vi "SetReference.vi"(8 "error in (no error)":errorcluster, 10 "Reference":string, 11 "Footnote in":refnum<class "FootnoteReference.lvclass">) -> (0 "error out":errorcluster, 3 "Footnote out":refnum<class "FootnoteReference.lvclass">)   [LabVIEW 2021, in "LvMarkdown.lvlib" / "FootnoteReference.lvclass"]
uses:
  FootnoteReference.lvclass
  FootnoteReference.lvclass/FootnoteReference.ctl
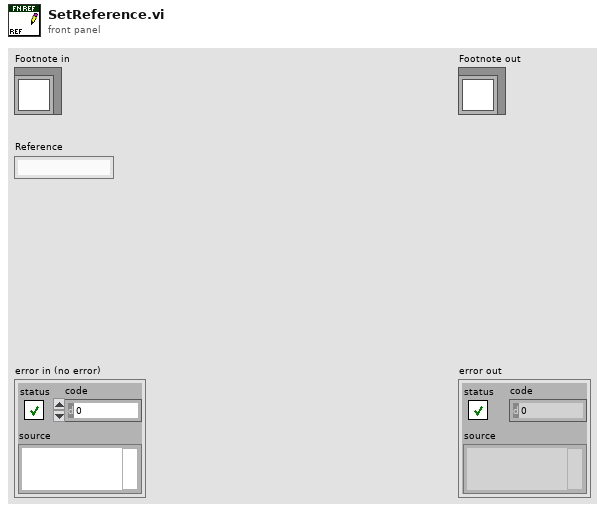
[diagram p1: front panel]
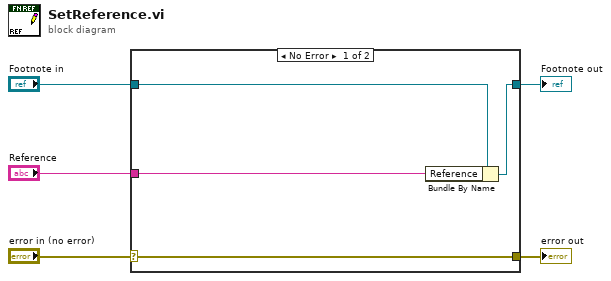
[diagram p0: block diagram]
diagram:
  n1 = case shown="No Error" "error in (no error)" {
    selector: "error in (no error)" -> [w9 w10]
    tunnel: [w9 w10] -> w4
    tunnel: [w7 w11] -> w2
    tunnel: "Footnote in" -> [w8 w11]
    tunnel: "Reference" -> [w6 _]
    frame No Error {
      n2 = Bundle By Name(cluster=w8, "Reference"=w6) -> (w7:refnum<class "FootnoteReference.lvclass">)
    }
    frame Error {
    }
  }
  "error out" <- w4
  "Footnote out" <- w2
